vi "setV_angSign.vi"(6 "current_dest":dbl[](array[numeric]) format="%#_13g", 7 "next_dest":dbl[](array[numeric]) format="%#_13g", 8 "error in (no error)":errorcluster, 9 "orientation":dbl format="%#_13g", 10 "v_ang":dbl format="%#_13g", 11 "Game in":refnum<class "Game.lvclass">) -> (0 "error out":errorcluster, 2 "v_ang_with_sign":dbl, 3 "Game out":refnum<class "Game.lvclass">)   [LabVIEW 2021, in "Game.lvclass"]
uses:
  Game.lvclass
  <vilib>/Analysis/coordinate.llb/Wrap Angle (scalar).vi
  <vilib>/Analysis/NI_AAL_Angle.lvlib
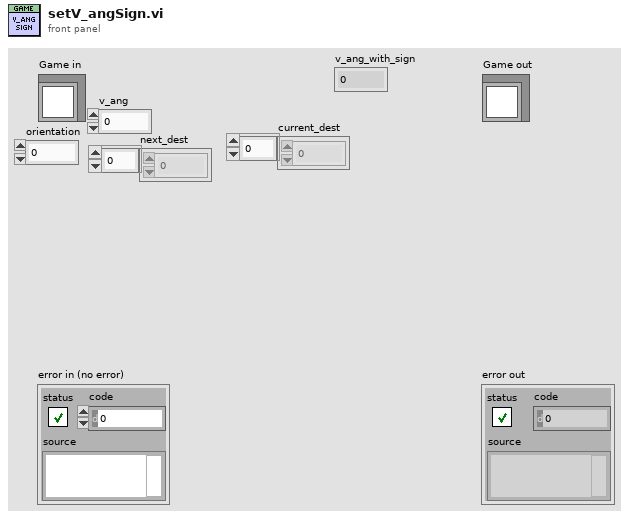
[diagram p1: front panel]
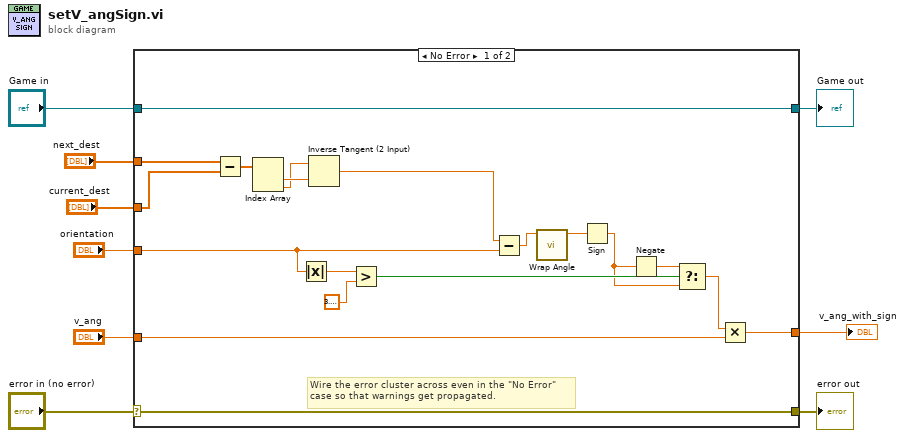
[diagram p0: block diagram]
diagram:
  n1 = case shown="No Error" "error in (no error)" {
    selector: "error in (no error)" -> [w27 w30]
    tunnel: [w27 w30] -> w8
    tunnel: [w28 w29] -> w6
    tunnel: "Game in" -> [w28 w29]
    tunnel: "orientation" -> [w23 _]
    tunnel: "current_dest" -> [w14 _]
    tunnel: "v_ang" -> [w18 _]
    tunnel: [w16 _] -> w2
    tunnel: "next_dest" -> [w15 _]
    frame No Error {
      # "Wire the error cluster across even in the \"No Error\"\ncase so that warnings get propagated."
      n2 = Subtract(x=w15, y=w14) -> (x-y=w13:dbl[])
      n3 = Index Array(array=w13) -> (element #1=w12:dbl, element #2=w11:dbl)  [unwired: 2 in]
      n4 = Absolute Value(x=w23) -> (abs(x)=w26:dbl)
      n5 = Inverse Tangent (2 Input)(1:w12, 2:w11) -> (0:w10:dbl)
      n6 = Greater?(x=w26, y=3.141592653589793) -> (0:w21:bool)
      n7 = Subtract(x=w10, y=w23) -> (x-y=w25:dbl)
      n8 = call-poly <vilib>:"Wrap Angle.vi"("angle in"=w25) -> ("angle out"=w22:dbl)  [unwired: 9 in, 1 out]
      n9 = Sign(1:w22) -> (0:w19:dbl)
      n10 = Negate(x=w19) -> (-x=w20:dbl)
      n11 = Select(t=w20, s=w21, f=w19) -> (s? t:f=w17:dbl)
      n12 = Multiply(x=w17, y=w18) -> (x*y=w16:dbl)
    }
    frame Error {
    }
  }
  "error out" <- w8
  "Game out" <- w6
  "v_ang_with_sign" <- w2
